vi "Server Connection Callback.vi"(7 "Owner":refnum<class>, 8 "error in (no error)":errorcluster, 9 "Data":variant, 10 "Connection State":T1, 11 "Connection":refnum<class "Connection.lvclass">) -> (0 "error out":errorcluster)   [LabVIEW 2020, in "Stream-Websocket.lvlib" / "Websocket Server.lvclass"]
uses:
  Websocket Server.lvclass
  Websocket Client/Websocket Client.lvclass
  lv-stream/stream/Connection/Connection.lvclass
  lv-stream/stream/Connection State.ctl
  lv-stream/stream/Stream.lvlib
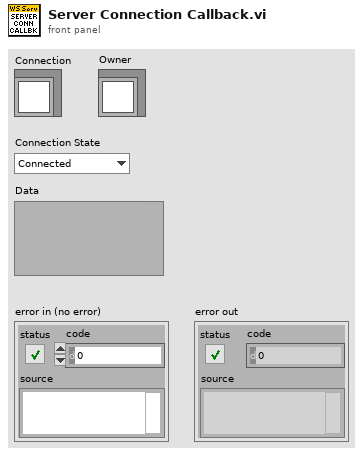
[diagram p1: front panel]
types:
  T1 = typedef "Stream.lvlib/Connection State.ctl" = enum16{"Connected", "Disconnected"}
  T2 = typedef "Stream-Websocket.lvlib/Websocket Server.lvclass/Ref Data.ctl" = cluster{"Listener":refnum<k5>, "Clients":refnum<class "Websocket Client.lvclass">[], "Open":bool}
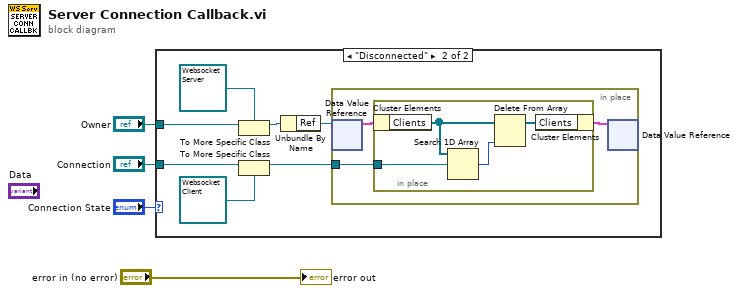
[diagram p0: block diagram]
diagram:
  n1 = case shown="\"Disconnected\"" "Connection State" {
    tunnel: "Owner" -> [_ w11]
    tunnel: "Connection" -> [_ w9]
    frame "Connected", Default {
    }
    frame "Disconnected" {
      n2 = To More Specific Class(target class=refnum<class "Websocket Server.lvclass"> refnum ("Stream-Websocket.lvlib:Websocket Server.lvclass"), reference=w11) -> (specific class reference=w6:refnum<class "Websocket Server.lvclass">)  [unwired: 1 in, 1 out]
      n3 = To More Specific Class(target class=refnum<class "Websocket Client.lvclass"> refnum ("Stream-Websocket.lvlib:Websocket Client.lvclass"), reference=w9) -> (specific class reference=w5:refnum<class "Websocket Client.lvclass">)  [unwired: 1 in, 1 out]
      n4 = Unbundle By Name(w6) -> ("Ref"=w7:refnum<data-value>)
      n5 = in-place {
        in-place-border: w5 -> [w12]
        n6 = in-place-dvr #1(w7) -> (w14:T2)  [unwired: 1 out]
        n7 = in-place {
          in-place-border: w12 -> [w18]
          n8 = in-place-cluster #2(w14) -> ("Clients"=w17:refnum<class "Websocket Client.lvclass">[])
          n9 = Search 1D Array(1D array=w17, element=w18) -> (index of element=w16:i32)  [unwired: 1 in]
          n10 = Delete From Array(array=w17, index=w16) -> (array with subset deleted=w15:refnum<class "Websocket Client.lvclass">[])  [unwired: 1 in, 1 out]
          n11 = in-place-cluster #2("Clients"=w15) -> (w13:T2)
        }
        n12 = in-place-dvr #1(w13) -> ()  [unwired: 2 out]
      }
    }
  }
  "error out" <- "error in (no error)"
